vi "AddTwoNumbers.vi"(3 "Numeric 2":dbl, 4 "Numeric 1":dbl, 5 ".NET Refnum":refnum<k24>) -> (0 "error out":errorcluster, 1 "Sum":dbl, 2 ".NET Refnum Out":refnum<k24>)   [LabVIEW 2010]
uses:
  \\camila\f$/Tests/LVBuildValidation/10.0/Automated/FlexLVAdapter30/Refnums/DotNetRefnum/LabviewDNTest.dll
  LabviewDNTest.dll
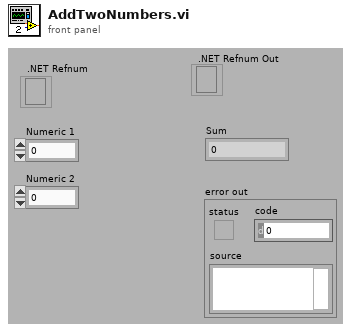
[diagram p1: front panel]
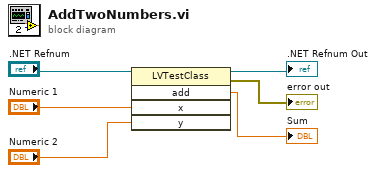
[diagram p0: block diagram]
diagram:
  n1 = invoke class="LVTestClass" method="add"(reference=".NET Refnum", "x"="Numeric 1", "y"="Numeric 2") -> (reference out=→".NET Refnum Out":refnum<k24>, error out=→"error out":errorcluster, "add"=→"Sum":dbl)  [unwired: 2 in, 2 out]
